vi "Toggle Discretes Mode.vi"(8 "error in":errorcluster, 10 "Discrete_Enable":bool, 11 "SL_SC in":refnum<class "SL_SC.lvclass">) -> (0 "error out":errorcluster, 3 "SL_SC out":refnum<class "SL_SC.lvclass">)   [LabVIEW 2019, in "SL_SC.lvlib" / "SL_SC.lvclass"]
uses:
  Library/SL_SC.lvclass
  Library/SL_SC.lvclass/SL_SC.ctl
  <vilib>/SLSC/Set Device Property (I32).vi
  <vilib>/SLSC/Commit Properties for Devices.vi
  <vilib>/SLSC/SLSC.lvlib
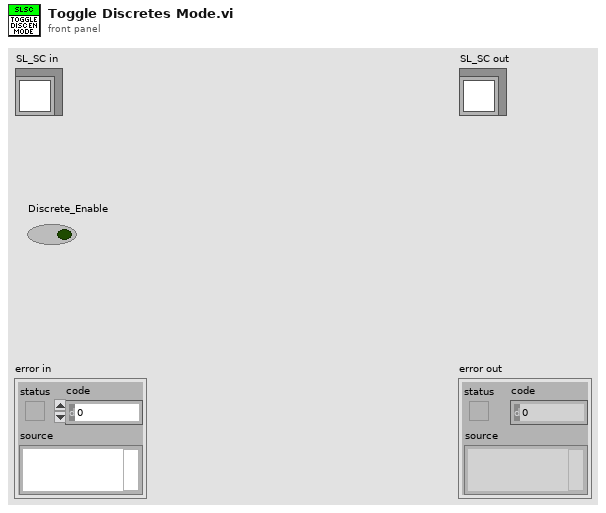
[diagram p1: front panel]
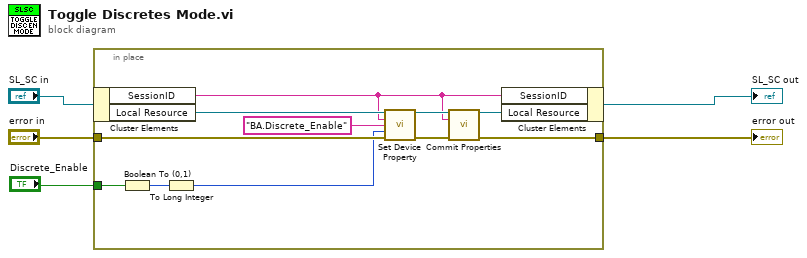
[diagram p0: block diagram]
diagram:
  n1 = in-place {
    in-place-border: "error in" -> [w15]
    in-place-border: [w7] -> w3
    in-place-border: "Discrete_Enable" -> [w14]
    n2 = in-place-cluster #1("SL_SC in") -> ("SessionID"=w6:string, "Local Resource"=w16:refnum<k21>)
    n3 = Boolean To (0,1)(Boolean=w14) -> (0, 1=w13:i16)
    n4 = To Long Integer(number=w13) -> (32bit integer=w12:i32)
    n5 = call-poly <vilib>:"Set Device Property.vi"("session in"=w16, "devices"=w6, "property"="BA.Discrete_Enable", "property value"=w12, "error in (no error)"=w15) -> ("session out"=w10:refnum<k21>, "error out"=w9:errorcluster)  [unwired: 9 in]
    n6 = call-poly <vilib>:"Commit Properties.vi"("session in"=w10, "devices"=w6, "error in (no error)"=w9) -> ("session out"=w8:refnum<k21>, "error out"=w7:errorcluster)  [unwired: 11 in]
    n7 = in-place-cluster #1("SessionID"=w6, "Local Resource"=w8) -> (→"SL_SC out":refnum<class "SL_SC.lvclass">)
  }
  "error out" <- w3
